vi "My_RIGOL_v1_1.vi"() -> ()   [LabVIEW 2012]
uses:
  RIGOL DG4000 Series.lvlib
panel:
  out "XY Graph":cluster{"Y":dbl[], "Y":dbl[]}[](graph)
  out "Выход на канал 2":string
  out "Выход на канал 1(тупиковый)":string
  out "String 8":string
  out "String 7":string
  out "String 6":string
  out "String 5":string caption="String"
  in  "Количество точек 2":dbl
  in  "Время между импульсами, с 2":dbl
  in  "Ширина импульса, с 2":dbl=1000.0
  out "String 4":string
  out "String 3":string
  out "String 2":string
  out "String":string
  in  "Количество точек":dbl
  in  "Время между импульсами, с":dbl
  in  "Ширина импульса, с":dbl=1000.0
  out "Выход на канал 2 (тупиковый)":string
  out "Выход на канал 1":string
  in  "Amplitude Unit (0: Vpp) 2":i32(ring) items=["Vpp", "Vrms", "dBm"]
  in  "Amplitude (5 Vpp) 2":dbl=5.0
  in  "Amplitude Unit (0: Vpp)":i32(ring) items=["Vpp", "Vrms", "dBm"]
  in  "Amplitude (5 Vpp)":dbl=5.0
  in  "Частота (1000 Hz)":dbl=1000.0
  in  "VISA resource name":refnum<visa-resource-name>
  # "Chanel 2"
  # "Chanel 1"
  # "ДИОД"
  # "ДЕТЕКТОР"
  # "ДЕТЕКТОР"
  # "ДИОД"
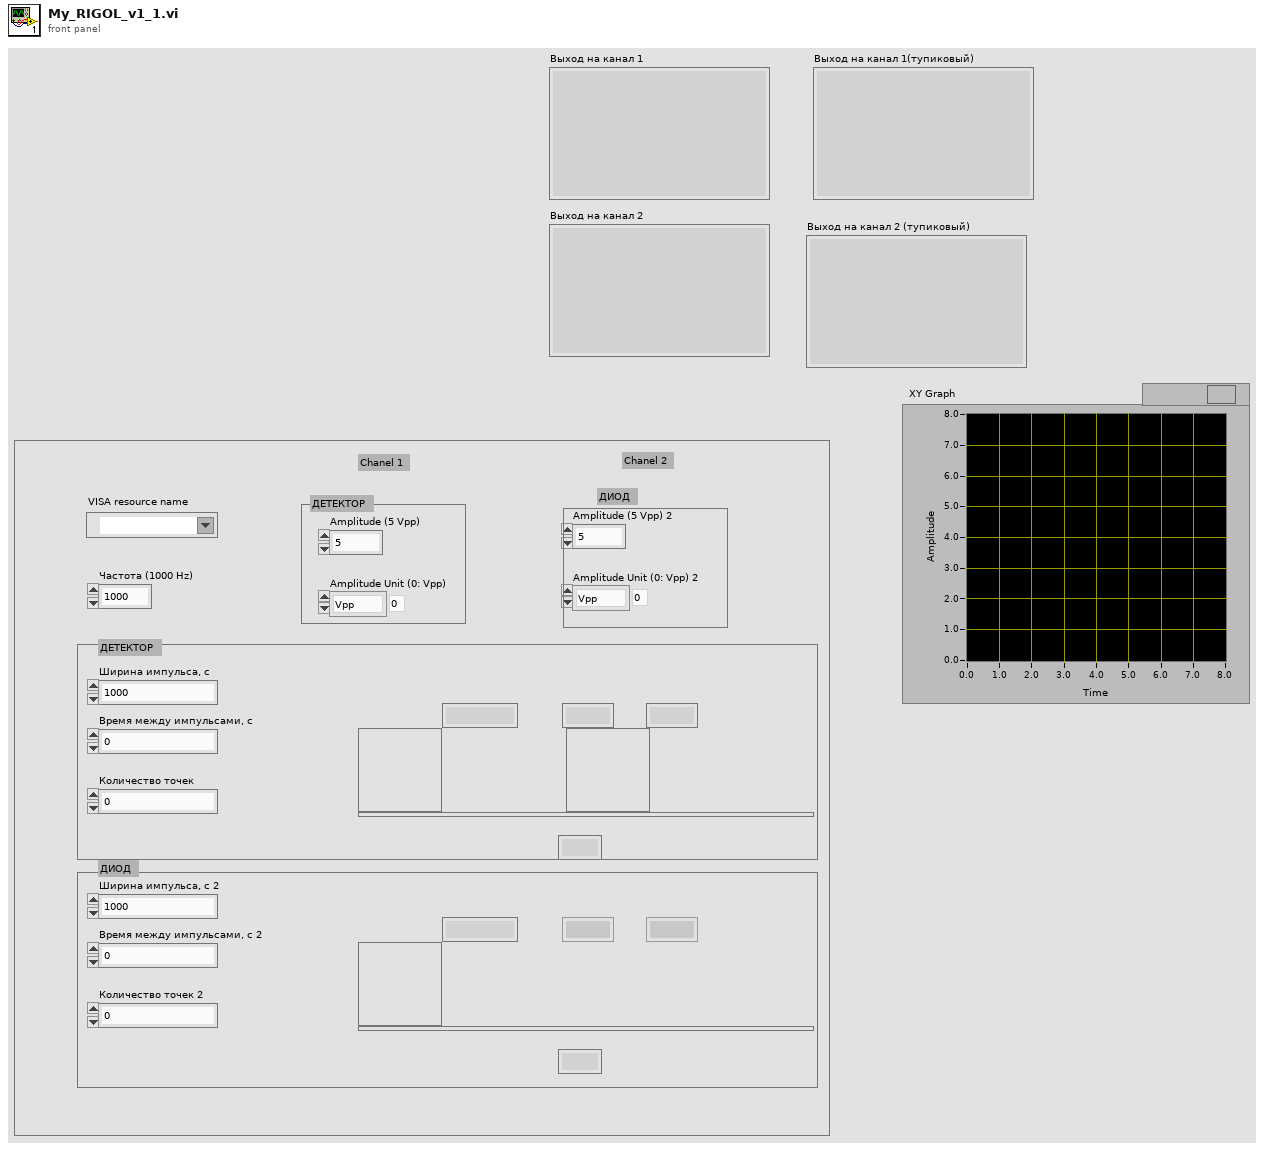
[diagram p1: front panel]
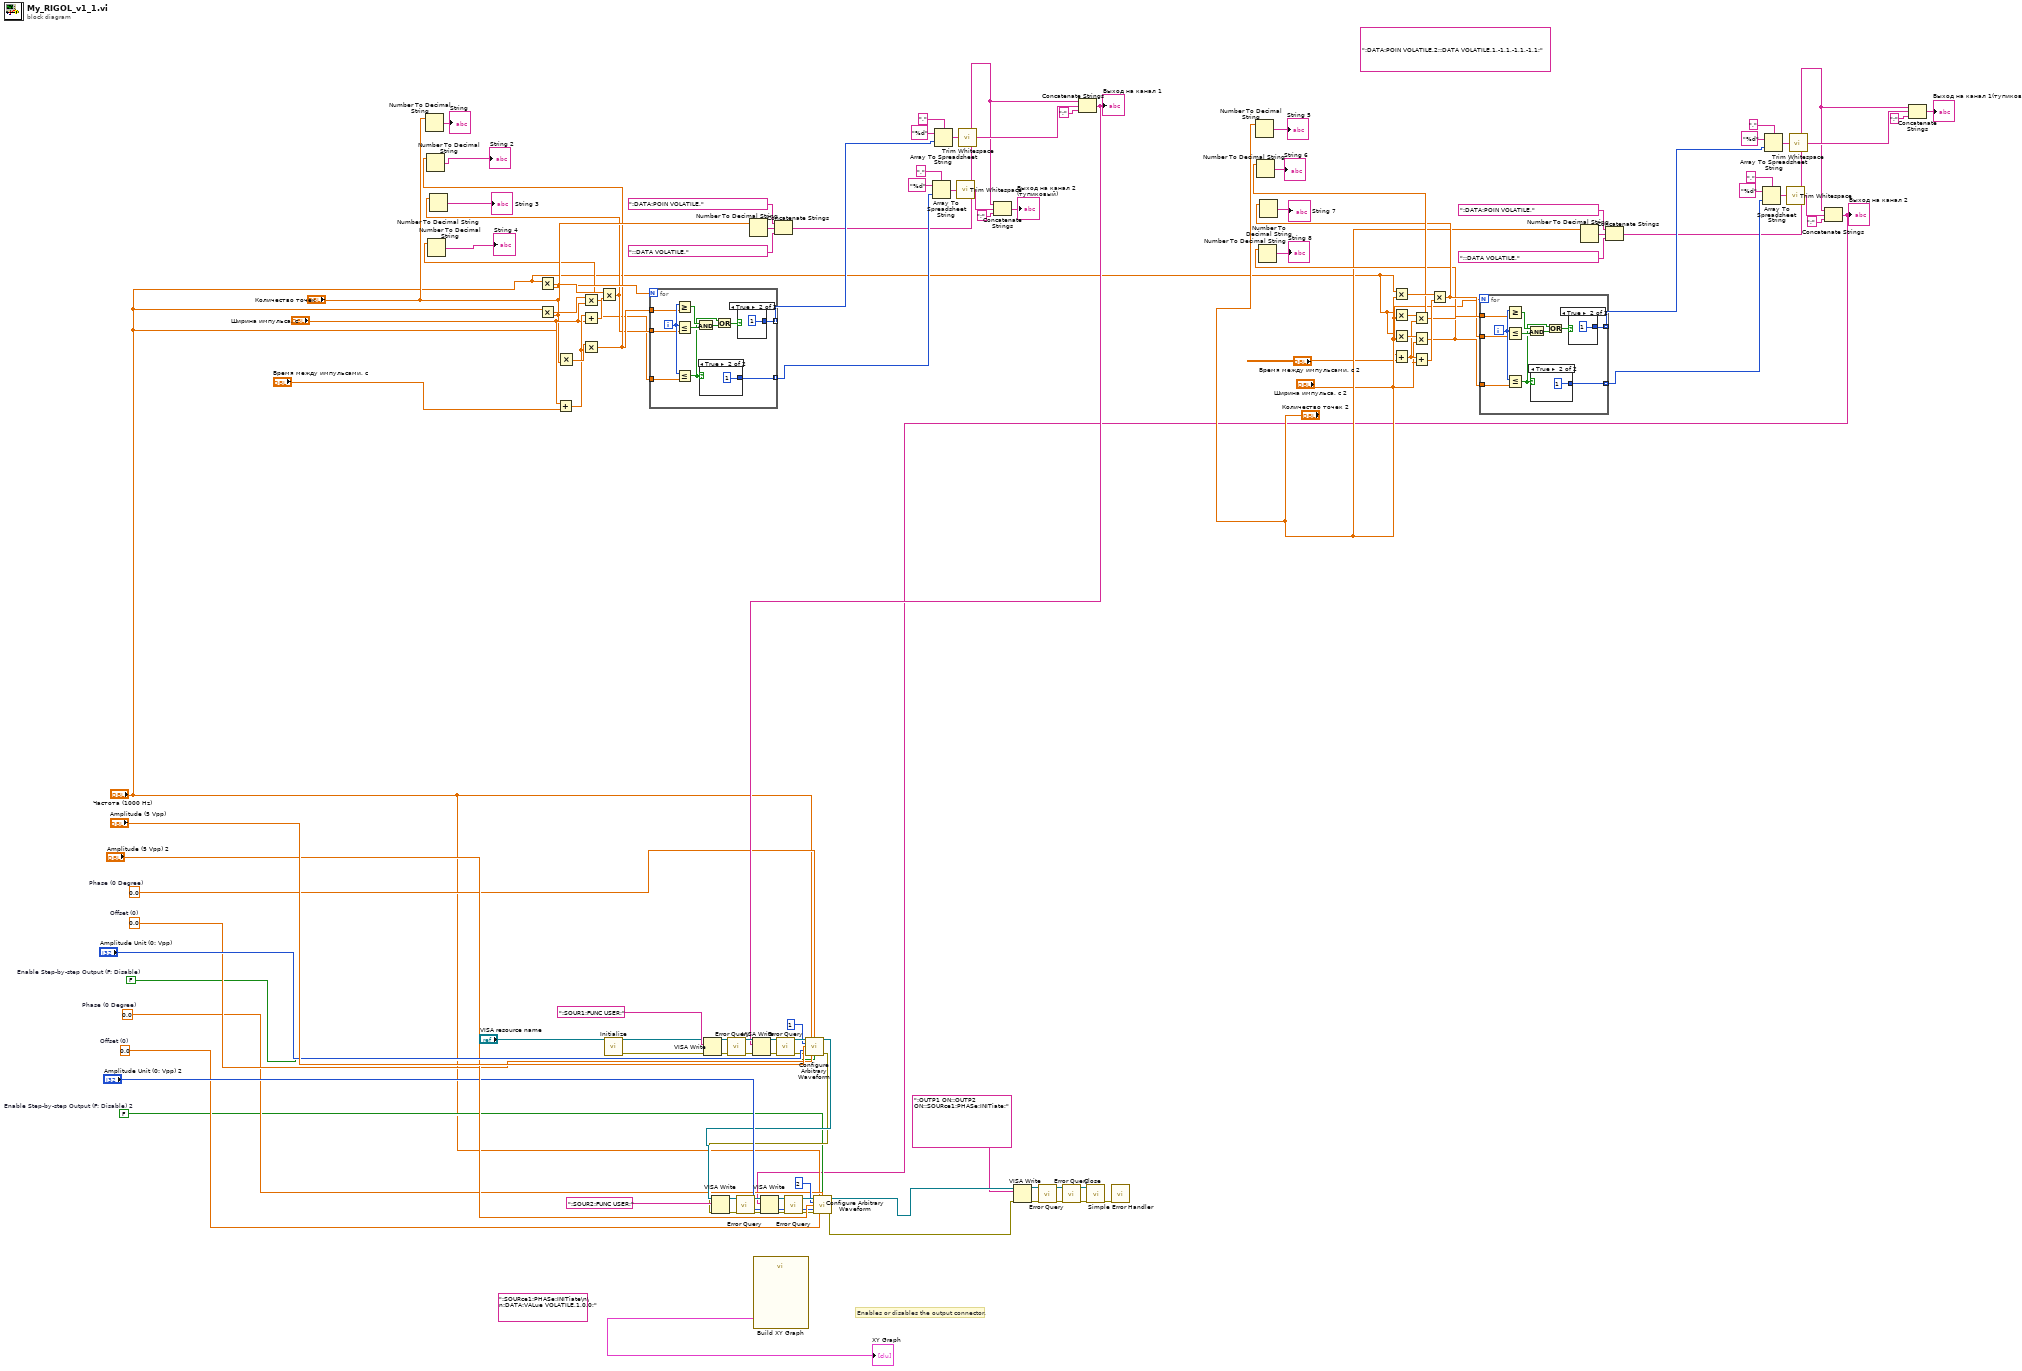
[diagram p0: block diagram]
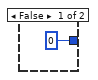
[diagram p2: hidden frame]
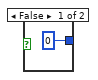
[diagram p3: hidden frame]
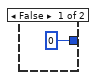
[diagram p4: hidden frame]
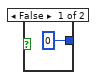
[diagram p5: hidden frame]
diagram:
  w39 = FALSE  # Enable Step-by-step Output (F: Disable) 2
  w40 = FALSE  # Enable Step-by-step Output (F: Disable)
  w41 = 0.0  # Offset (0)
  w42 = 0.0  # Phase (0 Degree)
  w43 = 0.0  # Offset (0)
  w44 = 0.0  # Phase (0 Degree)
  (unwired) ":SOURce1:PHASe:INITiate\n\n:DATA:VALue VOLATILE,1,0.0;"
  (unwired) ":DATA:POIN VOLATILE,2;:DATA VOLATILE,1,-1,1,-1,1,-1,1;"
  # "Enables or disables the output connector."
  n1 = Number To Decimal String(number="Количество точек") -> (decimal integer string=→"String":string)  [unwired: 1 in]
  n2 = Multiply(x="Частота (1000 Hz)", y="Количество точек") -> (x*y=w51:dbl)
  n3 = Multiply(x="Частота (1000 Hz)", y="Количество точек") -> (x*y=w56:dbl)
  n4 = Add(x="Ширина импульса, с", y="Время между импульсами, с") -> (x+y=w53:dbl)
  n5 = Multiply(x="Частота (1000 Hz)", y="Количество точек") -> (x*y=w55:dbl)
  n6 = Multiply(x=w56, y="Ширина импульса, с") -> (x*y=w45:dbl)
  n7 = Number To Decimal String(number=w45) -> (decimal integer string=→"String 4":string)  [unwired: 1 in]
  n8 = Add(x=w53, y="Ширина импульса, с") -> (x+y=w50:dbl)
  n9 = Multiply(x=w55, y=w53) -> (x*y=w47:dbl)
  n10 = Number To Decimal String(number=w47) -> (decimal integer string=→"String 2":string)  [unwired: 1 in]
  n11 = Multiply(x=w51, y=w50) -> (x*y=w46:dbl)
  n12 = Number To Decimal String(number=w46) -> (decimal integer string=→"String 3":string)  [unwired: 1 in]
  n13 = call "Initialize.vi"("VISA resource name"="VISA resource name") -> ("error out"=w84:errorcluster, "VISA resource name out"=w85:refnum<visa-resource-name>)  [unwired: 4 in, 5 out]
  n14 = for {
    N: "Количество точек" -> [_]
    tunnel: [w124] -> w72 mode=indexing
    tunnel: w45 -> [w123]
    tunnel: w47 -> [w117]
    tunnel: w46 -> [w116]
    tunnel: [w114] -> w65 mode=indexing
    i -> [w118]
    n15 = Greater Or Equal?(x=w118, y=w117) -> (x >= y?=w120:bool)
    n16 = Less Or Equal?(x=w118, y=w116) -> (x <= y?=w119:bool)
    n17 = Less Or Equal?(x=w118, y=w123) -> (x <= y?=w115:bool)
    n18 = And(x=w120, y=w119) -> (x .and. y?=w122:bool)
    n19 = case shown="True" w115 {
      tunnel: [0 1] -> w114
      frame False {
      }
      frame True {
      }
    }
    n20 = Or(x=w115, y=w122) -> (x .or. y?=w121:bool)
    n21 = case shown="True" w121 {
      tunnel: [0 1] -> w124
      frame False {
      }
      frame True {
      }
    }
  }
  n22 = VISA Write(VISA resource name=w85, write buffer=":SOUR1:FUNC USER;", error in (no error)=w84) -> (VISA resource name out=w109:refnum<visa-resource-name>, error out=w107:errorcluster)  [unwired: 1 out]
  n23 = call "Error Query.vi"("error in (no error)"=w107, "VISA resource name"=w109) -> ("error out"=w101:errorcluster, "VISA resource name out"=w104:refnum<visa-resource-name>)  [unwired: 8 out]
  n24 = Number To Decimal String(number="Количество точек") -> (decimal integer string=w62:string)  [unwired: 1 in]
  n25 = call "Build XY Graph"() -> ("XY Graph"=→"XY Graph":cluster{"Y":dbl[], "Y":dbl[]}[])  [unwired: 5 in, 6 out]
  n26 = Concatenate Strings(":DATA:POIN VOLATILE,", w62, ";:DATA VOLATILE,") -> (w59:string)
  n27 = Array To Spreadsheet String(delimiter (Tab)=",", array=w65, 3:"%d") -> (spreadsheet string=w67:string)
  n28 = Array To Spreadsheet String(delimiter (Tab)=",", array=w72, 3:"%d") -> (spreadsheet string=w73:string)
  n29 = call <vilib>:"Trim Whitespace.vi"("string"=w67) -> ("trimmed string"=w66:string)  [unwired: 1 in]
  n30 = call <vilib>:"Trim Whitespace.vi"("string"=w73) -> ("trimmed string"=w71:string)  [unwired: 1 in]
  n31 = Concatenate Strings(w59, w66, ";" ("delimiter (Tab)")) -> (→"Выход на канал 2 (тупиковый)":string)
  n32 = Concatenate Strings(w59, w71, ";" ("delimiter (Tab)")) -> (w63:string)
  "Выход на канал 1" <- w63
  n33 = VISA Write(VISA resource name=w104, write buffer=w63, error in (no error)=w101) -> (VISA resource name out=w103:refnum<visa-resource-name>, error out=w100:errorcluster)  [unwired: 1 out]
  n34 = call "Error Query.vi"("error in (no error)"=w100, "VISA resource name"=w103) -> ("error out"=w99:errorcluster, "VISA resource name out"=w102:refnum<visa-resource-name>)  [unwired: 8 out]
  n35 = call "Configure Arbitrary Waveform.vi"("VISA resource name"=w102, "Frequency (1000 Hz)"="Частота (1000 Hz)", "Phase (0 Degree)"=w44, "Output Channel (1: Channel 1)"=1, "Amplitude (5 Vpp)"="Amplitude (5 Vpp)", "Amplitude Unit (0: Vpp)"="Amplitude Unit (0: Vpp)", "error in (no error)"=w99, "Offset (0)"=w43, "Enable Step-by-step Output (F: Disable)"=w40) -> ("VISA resource name out"=w87:refnum<visa-resource-name>, "error out"=w86:errorcluster)  [unwired: 5 in]
  n36 = VISA Write(VISA resource name=w87, write buffer=":SOUR2:FUNC USER;", error in (no error)=w86) -> (VISA resource name out=w98:refnum<visa-resource-name>, error out=w96:errorcluster)  [unwired: 1 out]
  n37 = call "Error Query.vi"("error in (no error)"=w96, "VISA resource name"=w98) -> ("error out"=w90:errorcluster, "VISA resource name out"=w93:refnum<visa-resource-name>)  [unwired: 8 out]
  n38 = Number To Decimal String(number="Количество точек 2") -> (decimal integer string=→"String 5":string)  [unwired: 1 in]
  n39 = Multiply(x="Частота (1000 Hz)", y="Количество точек 2") -> (x*y=w18:dbl)
  n40 = Multiply(x="Частота (1000 Hz)", y="Количество точек 2") -> (x*y=w20:dbl)
  n41 = Multiply(x="Частота (1000 Hz)", y="Количество точек 2") -> (x*y=w21:dbl)
  n42 = Add(x="Ширина импульса, с 2", y="Время между импульсами, с 2") -> (x+y=w19:dbl)
  n43 = Multiply(x=w20, y=w19) -> (x*y=w16:dbl)
  n44 = Number To Decimal String(number=w16) -> (decimal integer string=→"String 6":string)  [unwired: 1 in]
  n45 = Multiply(x=w21, y="Ширина импульса, с 2") -> (x*y=w14:dbl)
  n46 = Number To Decimal String(number=w14) -> (decimal integer string=→"String 8":string)  [unwired: 1 in]
  n47 = Add(x=w19, y="Ширина импульса, с 2") -> (x+y=w17:dbl)
  n48 = Multiply(x=w18, y=w17) -> (x*y=w15:dbl)
  n49 = Number To Decimal String(number=w15) -> (decimal integer string=→"String 7":string)  [unwired: 1 in]
  n50 = for {
    N: "Количество точек 2" -> [_]
    tunnel: [w139] -> w34 mode=indexing
    tunnel: w14 -> [w138]
    tunnel: w16 -> [w132]
    tunnel: w15 -> [w131]
    tunnel: [w129] -> w27 mode=indexing
    i -> [w133]
    n51 = Greater Or Equal?(x=w133, y=w132) -> (x >= y?=w135:bool)
    n52 = Less Or Equal?(x=w133, y=w131) -> (x <= y?=w134:bool)
    n53 = Less Or Equal?(x=w133, y=w138) -> (x <= y?=w130:bool)
    n54 = And(x=w135, y=w134) -> (x .and. y?=w137:bool)
    n55 = case shown="True" w130 {
      tunnel: [0 1] -> w129
      frame False {
      }
      frame True {
      }
    }
    n56 = Or(x=w130, y=w137) -> (x .or. y?=w136:bool)
    n57 = case shown="True" w136 {
      tunnel: [0 1] -> w139
      frame False {
      }
      frame True {
      }
    }
  }
  n58 = Number To Decimal String(number="Количество точек 2") -> (decimal integer string=w25:string)  [unwired: 1 in]
  n59 = Concatenate Strings(":DATA:POIN VOLATILE,", w25, ";:DATA VOLATILE,") -> (w22:string)
  n60 = Array To Spreadsheet String(delimiter (Tab)=",", array=w27, 3:"%d") -> (spreadsheet string=w29:string)
  n61 = Array To Spreadsheet String(delimiter (Tab)=",", array=w34, 3:"%d") -> (spreadsheet string=w35:string)
  n62 = call <vilib>:"Trim Whitespace.vi"("string"=w29) -> ("trimmed string"=w28:string)  [unwired: 1 in]
  n63 = call <vilib>:"Trim Whitespace.vi"("string"=w35) -> ("trimmed string"=w33:string)  [unwired: 1 in]
  n64 = Concatenate Strings(w22, w28, ";" ("delimiter (Tab)")) -> (w5:string)
  "Выход на канал 2" <- w5
  n65 = VISA Write(VISA resource name=w93, write buffer=w5, error in (no error)=w90) -> (VISA resource name out=w92:refnum<visa-resource-name>, error out=w89:errorcluster)  [unwired: 1 out]
  n66 = call "Error Query.vi"("error in (no error)"=w89, "VISA resource name"=w92) -> ("error out"=w88:errorcluster, "VISA resource name out"=w91:refnum<visa-resource-name>)  [unwired: 8 out]
  n67 = call "Configure Arbitrary Waveform.vi"("VISA resource name"=w91, "Frequency (1000 Hz)"="Частота (1000 Hz)", "Phase (0 Degree)"=w42, "Output Channel (1: Channel 1)"=2, "Amplitude (5 Vpp)"="Amplitude (5 Vpp) 2", "Amplitude Unit (0: Vpp)"="Amplitude Unit (0: Vpp) 2", "error in (no error)"=w88, "Offset (0)"=w41, "Enable Step-by-step Output (F: Disable)"=w39) -> ("VISA resource name out"=w79:refnum<visa-resource-name>, "error out"=w78:errorcluster)  [unwired: 5 in]
  n68 = VISA Write(VISA resource name=w79, write buffer=":OUTP1 ON;:OUTP2 ON;:SOURce1:PHASe:INITiate;", error in (no error)=w78) -> (VISA resource name out=w81:refnum<visa-resource-name>, error out=w80:errorcluster)  [unwired: 1 out]
  n69 = call "Error Query.vi"("error in (no error)"=w80, "VISA resource name"=w81) -> ("error out"=w58:errorcluster, "VISA resource name out"=w57:refnum<visa-resource-name>)  [unwired: 8 out]
  n70 = call "Error Query.vi"("error in (no error)"=w58, "VISA resource name"=w57) -> ("error out"=w111:errorcluster, "VISA resource name out"=w112:refnum<visa-resource-name>)  [unwired: 8 out]
  n71 = call "Close.vi"("error in (no error)"=w111, "VISA resource name"=w112) -> ("error out"=w110:errorcluster)  [unwired: 9 out]
  n72 = call <vilib>:"Simple Error Handler.vi"("error in (no error)"=w110) -> ()  [unwired: 1 in, 8 out]
  n73 = Concatenate Strings(w22, w33, ";" ("delimiter (Tab)")) -> (→"Выход на канал 1(тупиковый)":string)
